vi "FIFO last element.vi"(8 "error in (no error)":errorcluster, 11 "Analog data":T1) -> (0 "error out":errorcluster, 1 "OK":bool, 2 "Last elements":dbl[](array[numeric]), 3 "Csatorna jellemzõk 2":T2[](array[typedef]))   [LabVIEW 2014]
uses:
  Analog data.ctl
panel:
  out "Array":i32[](array[numeric])
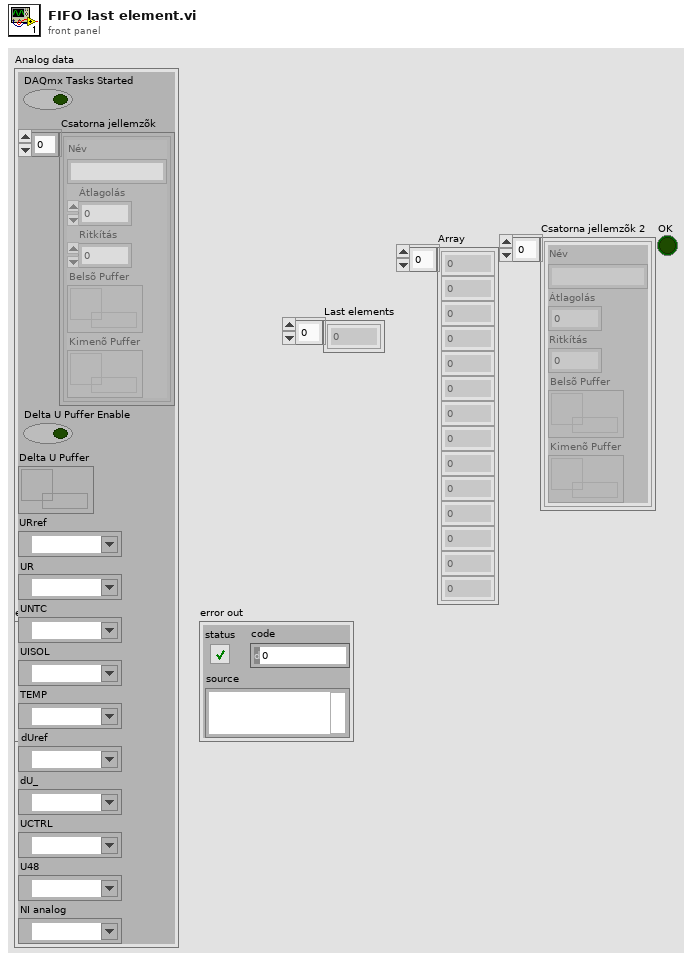
[diagram p1: front panel]
types:
  T1 = typedef "Analog data.ctl" = cluster{"DAQmx Tasks Started":bool, "Csatorna jellemzõk":T2[], "Delta U Puffer Enable":bool, "Delta U Puffer":refnum<queue>, "URref":refnum<k21>, "UR":refnum<k21>, "UNTC":refnum<k21>, "UISOL":refnum<k21>, "TEMP":refnum<k21>, "dUref":refnum<k21>, "dU_":refnum<k21>, "UCTRL":refnum<k21>, "U48":refnum<k21>, "NI analog":refnum<k21>}
  T2 = typedef "Csatorna jellemzõk.ctl" = cluster{"Név":string, "Átlagolás":i32, "Ritkítás":i32, "Belsõ Puffer":refnum<queue>, "Kimenõ Puffer":refnum<queue>}
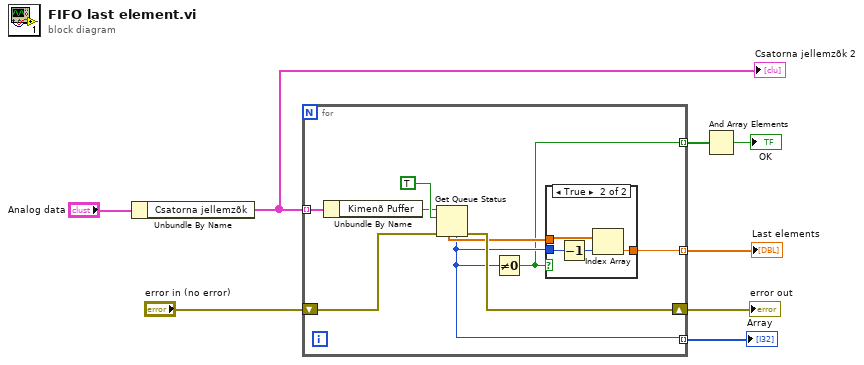
[diagram p0: block diagram]
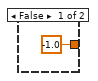
[diagram p2: hidden frame]
diagram:
  n1 = Unbundle By Name("Analog data") -> ("Csatorna jellemzõk"=w1:T2[])
  "Csatorna jellemzõk 2" <- w1
  n2 = for {
    tunnel: [w14] -> w6 mode=indexing
    tunnel: w1 -> [w11] mode=indexing
    shift-right: [w17] -> w8
    shift-left: "error in (no error)" -> [w16]
    tunnel: [w10] -> w5 mode=indexing
    tunnel: [w9] -> w4 mode=indexing
    n3 = Unbundle By Name(w11) -> ("Kimenõ Puffer"=w12:refnum<queue>)
    n4 = Get Queue Status(queue=w12, return elements? (F)=TRUE, error in (no error)=w16) -> (error out=w17:errorcluster, # elements in queue=w10:i32, elements=w13:dbl[])  [unwired: 5 out]
    n5 = Not Equal To 0?(x=w10) -> (x != 0?=w9:bool)
    n6 = case shown="True" w9 {
      tunnel: w13 -> [_ w22]
      tunnel: w10 -> [_ w20]
      tunnel: [-1.0 w19] -> w14
      frame False {
      }
      frame True {
        n7 = Decrement(x=w20) -> (x-1=w21:i32)
        n8 = Index Array(array=w22, index=w21) -> (element=w19:dbl)
      }
    }
  }
  "error out" <- w8
  "Last elements" <- w6
  "Array" <- w5
  n9 = And Array Elements(Boolean array=w4) -> (logical AND=→"OK":bool)
